vi "_Event Log.VerTest - Debug Util, Print to File.vi"() -> ()   [LabVIEW 2024, in "EQMF.lvlib" / "Event Log.lvlib"]
uses:
  Event Log.lvlib
panel:
  in  "Messages":string[](array[string])
  in  "Message":string
  in  "Enable Log":bool
  in  "stop":bool
  in  "OK Button":bool
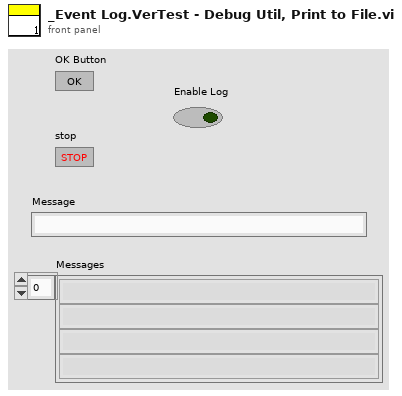
[diagram p1: front panel]
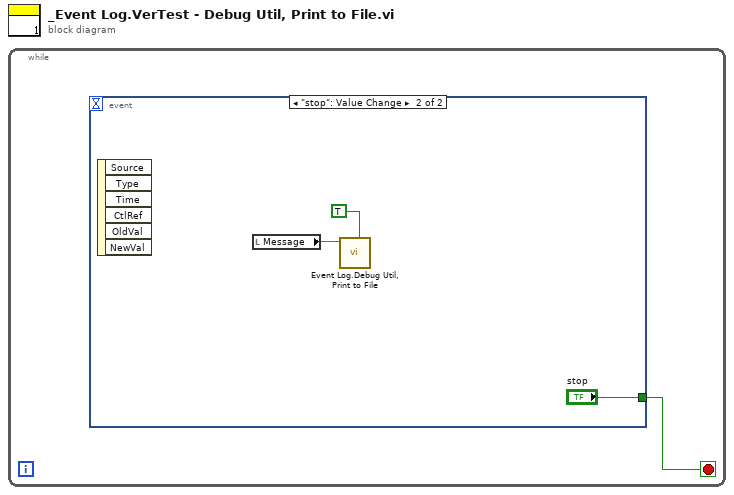
[diagram p0: block diagram]
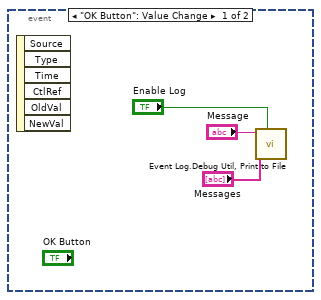
[diagram p2: hidden frame]
diagram:
  n1 = while {
    stop <- w1 stop-if-true
    n2 = event shown="[1] \"stop\": Value Change" {
      selector: _ -> [_ _]
      dyn-events: _ -> [_ _]
      timeout: _ -> [_ _]
      tunnel: [_ "stop"] -> w1
      event "OK Button": Value Change {
        n3 = event-data() -> ()  [unwired: 1 in, 6 out]
        n4 = call "Event Log.Debug Util, Print to File.vi"("Enable"="Enable Log", "Messages"="Messages", "Message"="Message") -> ()  [unwired: 9 in]
      }
      event "stop": Value Change {
        n5 = event-data() -> ()  [unwired: 1 in, 6 out]
        n6 = local read "Message"() -> (w5:string)
        n7 = call "Event Log.Debug Util, Print to File.vi"("Close"=TRUE, "Message"=w5) -> ()  [unwired: 10 in]
      }
    }
  }
